vi "rep_cap_pack.vi"(3 "RepCapName CmdValues":string[](array[string]), 5 "RepCapName IDs":string[](array[string])) -> (0 "Type out":i32(ring) items=["Arbitrary", "SequentialNull", "Sequential"], 2 "RepCap IDs out":variant)   [LabVIEW 2014, in "rszvl_rsidr_core.lvlib"]
uses:
  rszvl_rsidr_core.lvlib
  whitespace.ctl
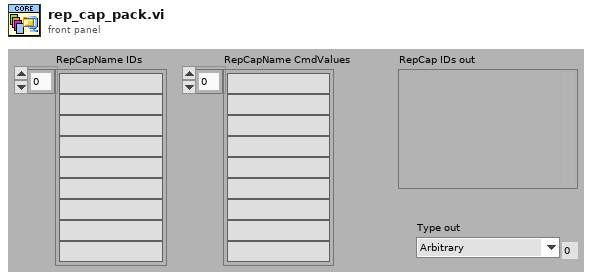
[diagram p1: front panel]
types:
  T1 = typedef "whitespace.ctl" = u16
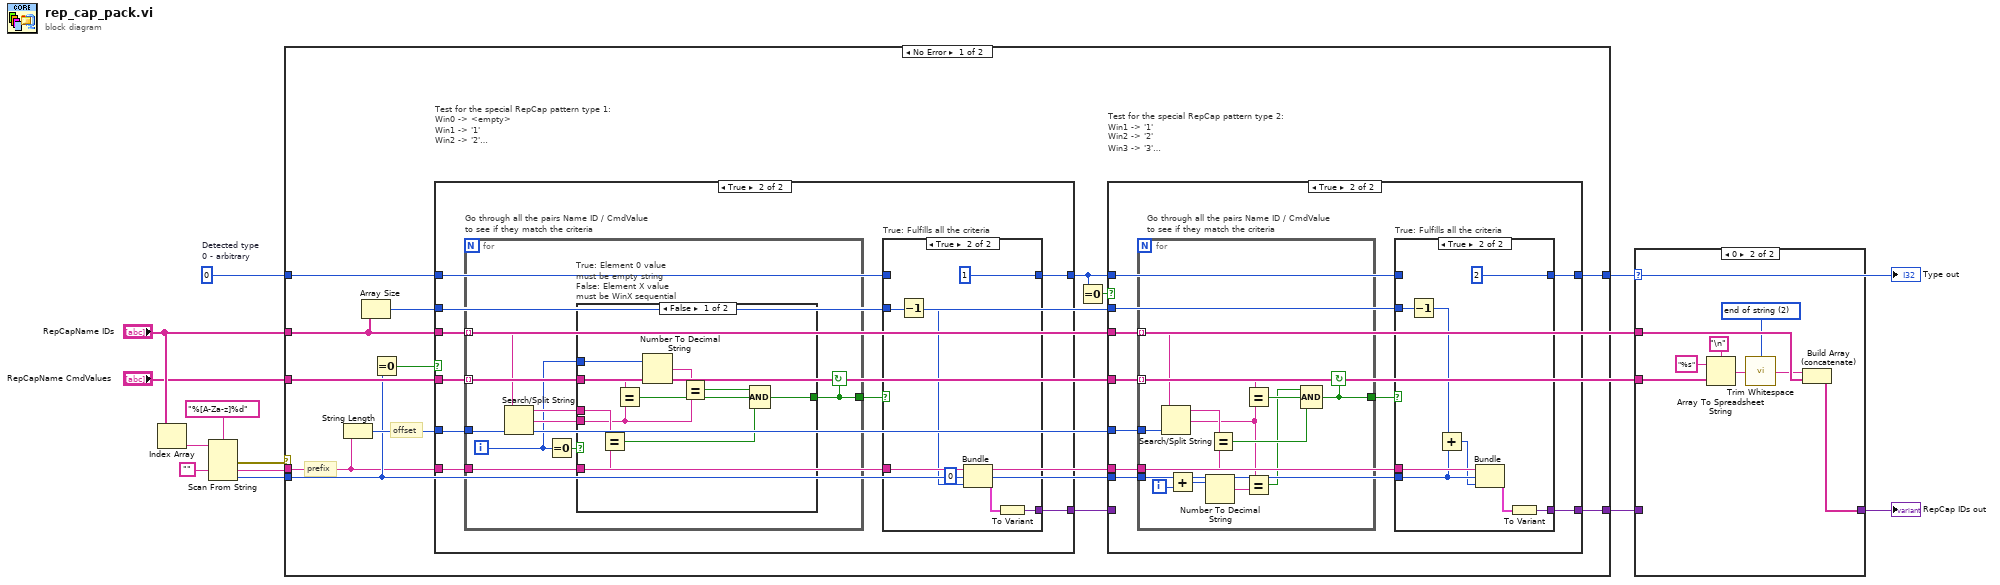
[diagram p0: block diagram]
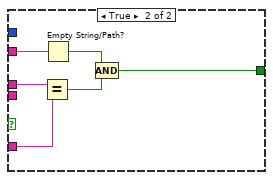
[diagram p7: hidden frame]
diagram:
  w5 = 0  # Detected type 0 - arbitrary
  n1 = Index Array(array="RepCapName IDs") -> (element=w12:string)  [unwired: 1 in]
  n2 = Scan From String(format string="%[A-Za-z]%d" ("string"), input string=w12, default 1="" ("Empty String Constant")) -> (error out=w10:errorcluster, output 1=w4:string, output 2=w3:i32)  [unwired: 3 in, 2 out]
  n3 = case shown="No Error" w10 {
    tunnel: "RepCapName IDs" -> [w16 _]
    tunnel: "RepCapName CmdValues" -> [w23 _]
    tunnel: w4 -> [w20 _]
    tunnel: w3 -> [w21 _]
    tunnel: w5 -> [w24 w104]
    tunnel: [w14 w104] -> w1
    tunnel: [w13 _] -> w2
    frame No Error {
      # "offset"
      # "prefix"
      n4 = String Length(string=w20) -> (length=w22:i32)
      n5 = Array Size(array=w16) -> (size(s)=w15:i32)
      n6 = Equal To 0?(x=w21) -> (x = 0?=w25:bool)
      n7 = case "Test for the special RepCap pattern type 1:\nWin0 -> <empty>\nWin1 -> '1'\nWin2 -> '2'\n\nName IDs must start with Win0 and the first CmdValue must be empty\nFor all the further NameIDs WinX the value must be X\nX values must be sequential, without an interruption" shown="True" w25 {
        tunnel: w16 -> [_ w70]
        tunnel: w23 -> [_ w69]
        tunnel: w24 -> [w61 w65]
        tunnel: w22 -> [_ w68]
        tunnel: [w61 w64] -> w18
        tunnel: w20 -> [_ w66]
        tunnel: [_ w63] -> w17
        tunnel: w15 -> [_ w62]
        frame False {
        }
        frame True {
          n8 = for "Go through all the pairs Name ID / CmdValue\nto see if they match the criteria" {
            tunnel: w70 -> [w84] mode=indexing
            tunnel: w69 -> [w87] mode=indexing
            tunnel: w66 -> [w85]
            tunnel: w68 -> [w83]
            tunnel: [w80] -> w67
            i -> [w79]
            stop <- w80 continue-if-true
            n9 = Search/Split String(string=w84, offset (0)=w83) -> (substring before match=w82:string, match + rest of string=w81:string)  [unwired: 1 in, 1 out]
            n10 = Equal To 0?(x=w79) -> (x = 0?=w86:bool)
            n11 = case "True: Element 0 value must be empty string\nFalse: Element X value must be WinX sequential" shown="False" w86 {
              tunnel: w87 -> [w96 w103]
              tunnel: w85 -> [w97 w101]
              tunnel: w79 -> [w93 _]
              tunnel: w82 -> [w91 w102]
              tunnel: w81 -> [w90 _]
              tunnel: [w88 w98] -> w80
              frame False {
                n12 = Equal?(x=w91, y=w97) -> (x = y?=w95:bool)
                n13 = Equal?(x=w96, y=w90) -> (x = y?=w94:bool)
                n14 = Number To Decimal String(number=w93) -> (decimal integer string=w92:string)  [unwired: 1 in]
                n15 = Equal?(x=w92, y=w90) -> (x = y?=w89:bool)
                n16 = Compound Arithmetic op=AND(w89, w94, w95) -> (w88:bool)
              }
              frame True {
                n17 = Equal?(x=w102, y=w101) -> (x = y?=w100:bool)
                n18 = Empty String/Path?(string/path=w103) -> (empty?=w99:bool)
                n19 = Compound Arithmetic op=AND(w99, w100) -> (w98:bool)
              }
            }
          }
          n20 = case "True: Fulfills all the criteria" shown="True" w67 {
            tunnel: w66 -> [_ w78]
            tunnel: w65 -> [w71 _]
            tunnel: [w71 1 ("Detected type\n0 - arbitrary")] -> w64
            tunnel: [_ w77] -> w63
            tunnel: w62 -> [_ w72]
            frame False {
            }
            frame True {
              n21 = Decrement(x=w72) -> (x-1=w73:i32)
              n22 = Bundle(w78, 0, w73) -> (w76:cluster{string, i32, i32})  [unwired: 1 in]
              n23 = To Variant(anything=w76) -> (Variant=w77:variant)
            }
          }
        }
      }
      n24 = Equal To 0?(x=w18) -> (x = 0?=w19:bool)
      n25 = case "Test for the special RepCap pattern type 2:\nWin1 -> '1'\nWin2 -> '2'\nWin3 -> '3'\n\nFor all the NameIDs WinX the value must be X\nX values must be sequential, without an interruption" shown="True" w19 {
        tunnel: w16 -> [_ w37]
        tunnel: w23 -> [_ w36]
        tunnel: w20 -> [_ w33]
        tunnel: w18 -> [w27 w28]
        tunnel: w22 -> [_ w35]
        tunnel: [w27 w29] -> w14
        tunnel: w21 -> [_ w31]
        tunnel: w17 -> [w26 _]
        tunnel: [w26 w30] -> w13
        tunnel: w15 -> [_ w32]
        frame False {
        }
        frame True {
          n26 = for "Go through all the pairs Name ID / CmdValue\nto see if they match the criteria" {
            tunnel: w37 -> [w58] mode=indexing
            tunnel: w36 -> [w60] mode=indexing
            tunnel: w33 -> [w59]
            tunnel: w35 -> [w57]
            tunnel: [w55] -> w34
            tunnel: w31 -> [w51]
            i -> [w50]
            stop <- w55 continue-if-true
            n27 = Search/Split String(string=w58, offset (0)=w57) -> (substring before match=w56:string, match + rest of string=w48:string)  [unwired: 1 in, 1 out]
            n28 = Add(x=w51, y=w50) -> (x+y=w47:i32)
            n29 = Number To Decimal String(number=w47) -> (decimal integer string=w49:string)  [unwired: 1 in]
            n30 = Equal?(x=w56, y=w59) -> (x = y?=w54:bool)
            n31 = Equal?(x=w60, y=w48) -> (x = y?=w53:bool)
            n32 = Equal?(x=w48, y=w49) -> (x = y?=w52:bool)
            n33 = Compound Arithmetic op=AND(w52, w53, w54) -> (w55:bool)
          }
          n34 = case "True: Fulfills all the criteria" shown="True" w34 {
            tunnel: w33 -> [_ w46]
            tunnel: [w38 2 ("Detected type\n0 - arbitrary")] -> w29
            tunnel: [_ w45] -> w30
            tunnel: w32 -> [_ w42]
            tunnel: w31 -> [_ w41]
            tunnel: w28 -> [w38 _]
            frame False {
            }
            frame True {
              n35 = Decrement(x=w42) -> (x-1=w39:i32)
              n36 = Add(x=w39, y=w41) -> (x+y=w40:i32)
              n37 = Bundle(w46, w41, w40) -> (w44:cluster{string, i32, i32})  [unwired: 1 in]
              n38 = To Variant(anything=w44) -> (Variant=w45:variant)
            }
          }
        }
      }
    }
    frame Error {
    }
  }
  "Type out" <- w1
  n39 = case shown="0" w1 {
    tunnel: w2 -> [w105 _]
    tunnel: "RepCapName IDs" -> [_ w109]
    tunnel: "RepCapName CmdValues" -> [_ w113]
    tunnel: [w105 w108] -> w6
    frame 1, Default {
    }
    frame 0 {
      w106 = T1 2 items=["both", "start of string", "end of string"] ("location (both)")
      n40 = Array To Spreadsheet String(delimiter (Tab)="\n" ("Line Feed Constant"), array=w113, 3:"%s" ("format string")) -> (spreadsheet string=w110:string)
      n41 = call "Trim Whitespace.vi"("string"=w110, "location (both)"=w106) -> ("trimmed string"=w107:string)
      n42 = Build Array (concatenate)(w107, w109) -> (w108:string[])
    }
  }
  "RepCap IDs out" <- w6
